vi "WriteReadRegisterLambdaSIM.vi"(4 "period":dbl[](array[numeric]), 5 "VS feedback":dbl[](array[numeric]), 6 "devices 2":refnum<k21>="SLSC-12001-0310EC4F-Mod4", 7 "par 3":T1={"Loop time"={"Loop Rate"=5, "Processor"=-2}, "COM"={"COM IP"="192.168.8.70", "COM port"=30005, "Local port"=5556, "Next_IP 1"=0, "Next_IP 2"=0, "Next_IP 3"=0, "Next_IP 4"=0}, "O2Sensor1"={"Lambda"={"LSU4.2 Lambda"=[], "LSU4.2 Ip"=[], "LSU4.9 Lambda"=[], "LSU4.9 Ip"=[], "LZA03 Lambda"=[], "LZA03 Ip"=[], "LZA08 Lambda"=[], "LZA08 Ip"=[], "Custom Lambda"=[], "Custom Ip"=[]}, "Temp"={"LSU4.2 Temp"=[], "LSU4.2 Ohm"=[], "LSU4.9 Temp"=[], "LSU4.9 Ohm"=[], "LZA03 Temp"=[], "LZA03 Ohm"=[], "LZA08 Temp"=[], "LZA08 Ohm"=[], "Custom Temp"=[], "Custom Ohm"=[]}, "Lambda Type"=0, "PID"={"Ki"=0.0, "Kp"=0.0, "Kd"=0.0, "FeedFW"=0.0}}, "O2Sensor2"={"Lambda"={"LSU4.2 Lambda"=[], "LSU4.2 Ip"=[], "LSU4.9 Lambda"=[], "LSU4.9 Ip"=[], "LZA03 Lambda"=[], "LZA03 Ip"=[], "LZA08 Lambda"=[], "LZA08 Ip"=[], "Custom Lambda"=[], "Custom Ip"=[]}, "Temp"={"LSU4.2 Temp"=[], "LSU4.2 Ohm"=[], "LSU4.9 Temp"=[], "LSU4.9 Ohm"=[], "LZA03 Temp"=[], "LZA03 Ohm"=[], "LZA08 Temp"=[], "LZA08 Ohm"=[], "Custom Temp"=[], "Custom Ohm"=[]}, "Lambda Type"=0, "PID"={"Ki"=0.0, "Kp"=0.0, "Kd"=0.0, "FeedFW"=0.0}}, "O2Sensor3"={"Lambda"={"LSU4.2 Lambda"=[], "LSU4.2 Ip"=[], "LSU4.9 Lambda"=[], "LSU4.9 Ip"=[], "LZA03 Lambda"=[], "LZA03 Ip"=[], "LZA08 Lambda"=[], "LZA08 Ip"=[], "Custom Lambda"=[], "Custom Ip"=[]}, "Temp"={"LSU4.2 Temp"=[], "LSU4.2 Ohm"=[], "LSU4.9 Temp"=[], "LSU4.9 Ohm"=[], "LZA03 Temp"=[], "LZA03 Ohm"=[], "LZA08 Temp"=[], "LZA08 Ohm"=[], "Custom Temp"=[], "Custom Ohm"=[]}, "Lambda Type"=0, "PID"={"Ki"=0.0, "Kp"=0.0, "Kd"=0.0, "FeedFW"=0.0}}, "O2Sensor4"={"Lambda"={"LSU4.2 Lambda"=[], "LSU4.2 Ip"=[], "LSU4.9 Lambda"=[], "LSU4.9 Ip"=[], "LZA03 Lambda"=[], "LZA03 Ip"=[], "LZA08 Lambda"=[], "LZA08 Ip"=[], "Custom Lambda"=[], "Custom Ip"=[]}, "Temp"={"LSU4.2 Temp"=[], "LSU4.2 Ohm"=[], "LSU4.9 Temp"=[], "LSU4.9 Ohm"=[], "LZA03 Temp"=[], "LZA03 Ohm"=[], "LZA08 Temp"=[], "LZA08 Ohm"=[], "Custom Temp"=[], "Custom Ohm"=[]}, "Lambda Type"=0, "PID"={"Ki"=0.0, "Kp"=0.0, "Kd"=0.0, "FeedFW"=0.0}}, "Board"=0, "Mode"=enum."SLSC Mode", "vendor.Num"=4141, "product.Num"=0} {"Board" items=["O2Sim_2ch", "O2Sim_4ch"]; "O2Sensor4"."Lambda Type" items=["LSU4.2", "LSU4.9", "LZA03", "LZA08", "Custom", "[mA]"]; "O2Sensor3"."Lambda Type" items=["LSU4.2", "LSU4.9", "LZA03", "LZA08", "Custom", "[mA]"]; "O2Sensor2"."Lambda Type" items=["LSU4.2", "LSU4.9", "LZA03", "LZA08", "Custom", "[mA]"]; "O2Sensor1"."Lambda Type" items=["LSU4.2", "LSU4.9", "LZA03", "LZA08", "Custom", "[mA]"]}, 8 "error in":errorcluster, 9 "SensorUsed":T3, 10 "VS Control":dbl[](array[numeric]), 11 "session in":refnum<k21>) -> (0 "error out":errorcluster, 2 "VS feedback":dbl[](array[numeric]), 3 "session out":refnum<k21>)   [LabVIEW 2017, in "ALMA_10201-10401_O2SensorSim Engine.lvlib"]
uses:
  ALMA_10201-10401_O2SensorSim Engine.lvlib
  Sensor_used.ctl
  Par.ctl
  LambdaType.ctl
  <vilib>/SLSC/Write Register (U64).vi
  <vilib>/SLSC/Read Register (U64).vi
  <vilib>/SLSC/Set Device Property (I32).vi
  <vilib>/SLSC/SLSC.lvlib
panel:
  out "element":dbl(graph)
  out "#ch_choise":enum16{"O2Sim_2ch", "O2Sim_4ch"}(ring)
  out "com error out":bool
  out "Status":bool[](array[boolean])
  out "Heater DC Indicator":u8[](array[numeric])=[64, 15, 32, 16]
  out "Heater Frequency Indicator2":u8[](array[numeric])=[128, 190, 128, 220]
  out "IP Feedback":dbl[](array[numeric])
  out "Command Cunter Feedback":u8=255
  out "Program Running Cunter":u8=96
  out "IP Feedback 7":dbl[](array[numeric])
  out "Command Cunter Feedback 7":u8=255
  out "Program Running Cunter 7":u8=96
  in  "CommandData 7":u64 format="%048b"
  out "IP Feedback 6":dbl[](array[numeric])
  out "Command Cunter Feedback 6":u8=255
  out "Program Running Cunter 6":u8=96
  in  "CommandData 6":u64 format="%048b"
  out "IP Feedback 5":dbl[](array[numeric])
  out "Command Cunter Feedback 5":u8=255
  out "Program Running Cunter 5":u8=96
  in  "CommandData 5":u64 format="%048b"
  out "IP Feedback 3":dbl[](array[numeric])
  out "Command Cunter Feedback 3":u8=255
  out "Program Running Cunter 3":u8=96
  in  "CommandData 3":u64 format="%048b"
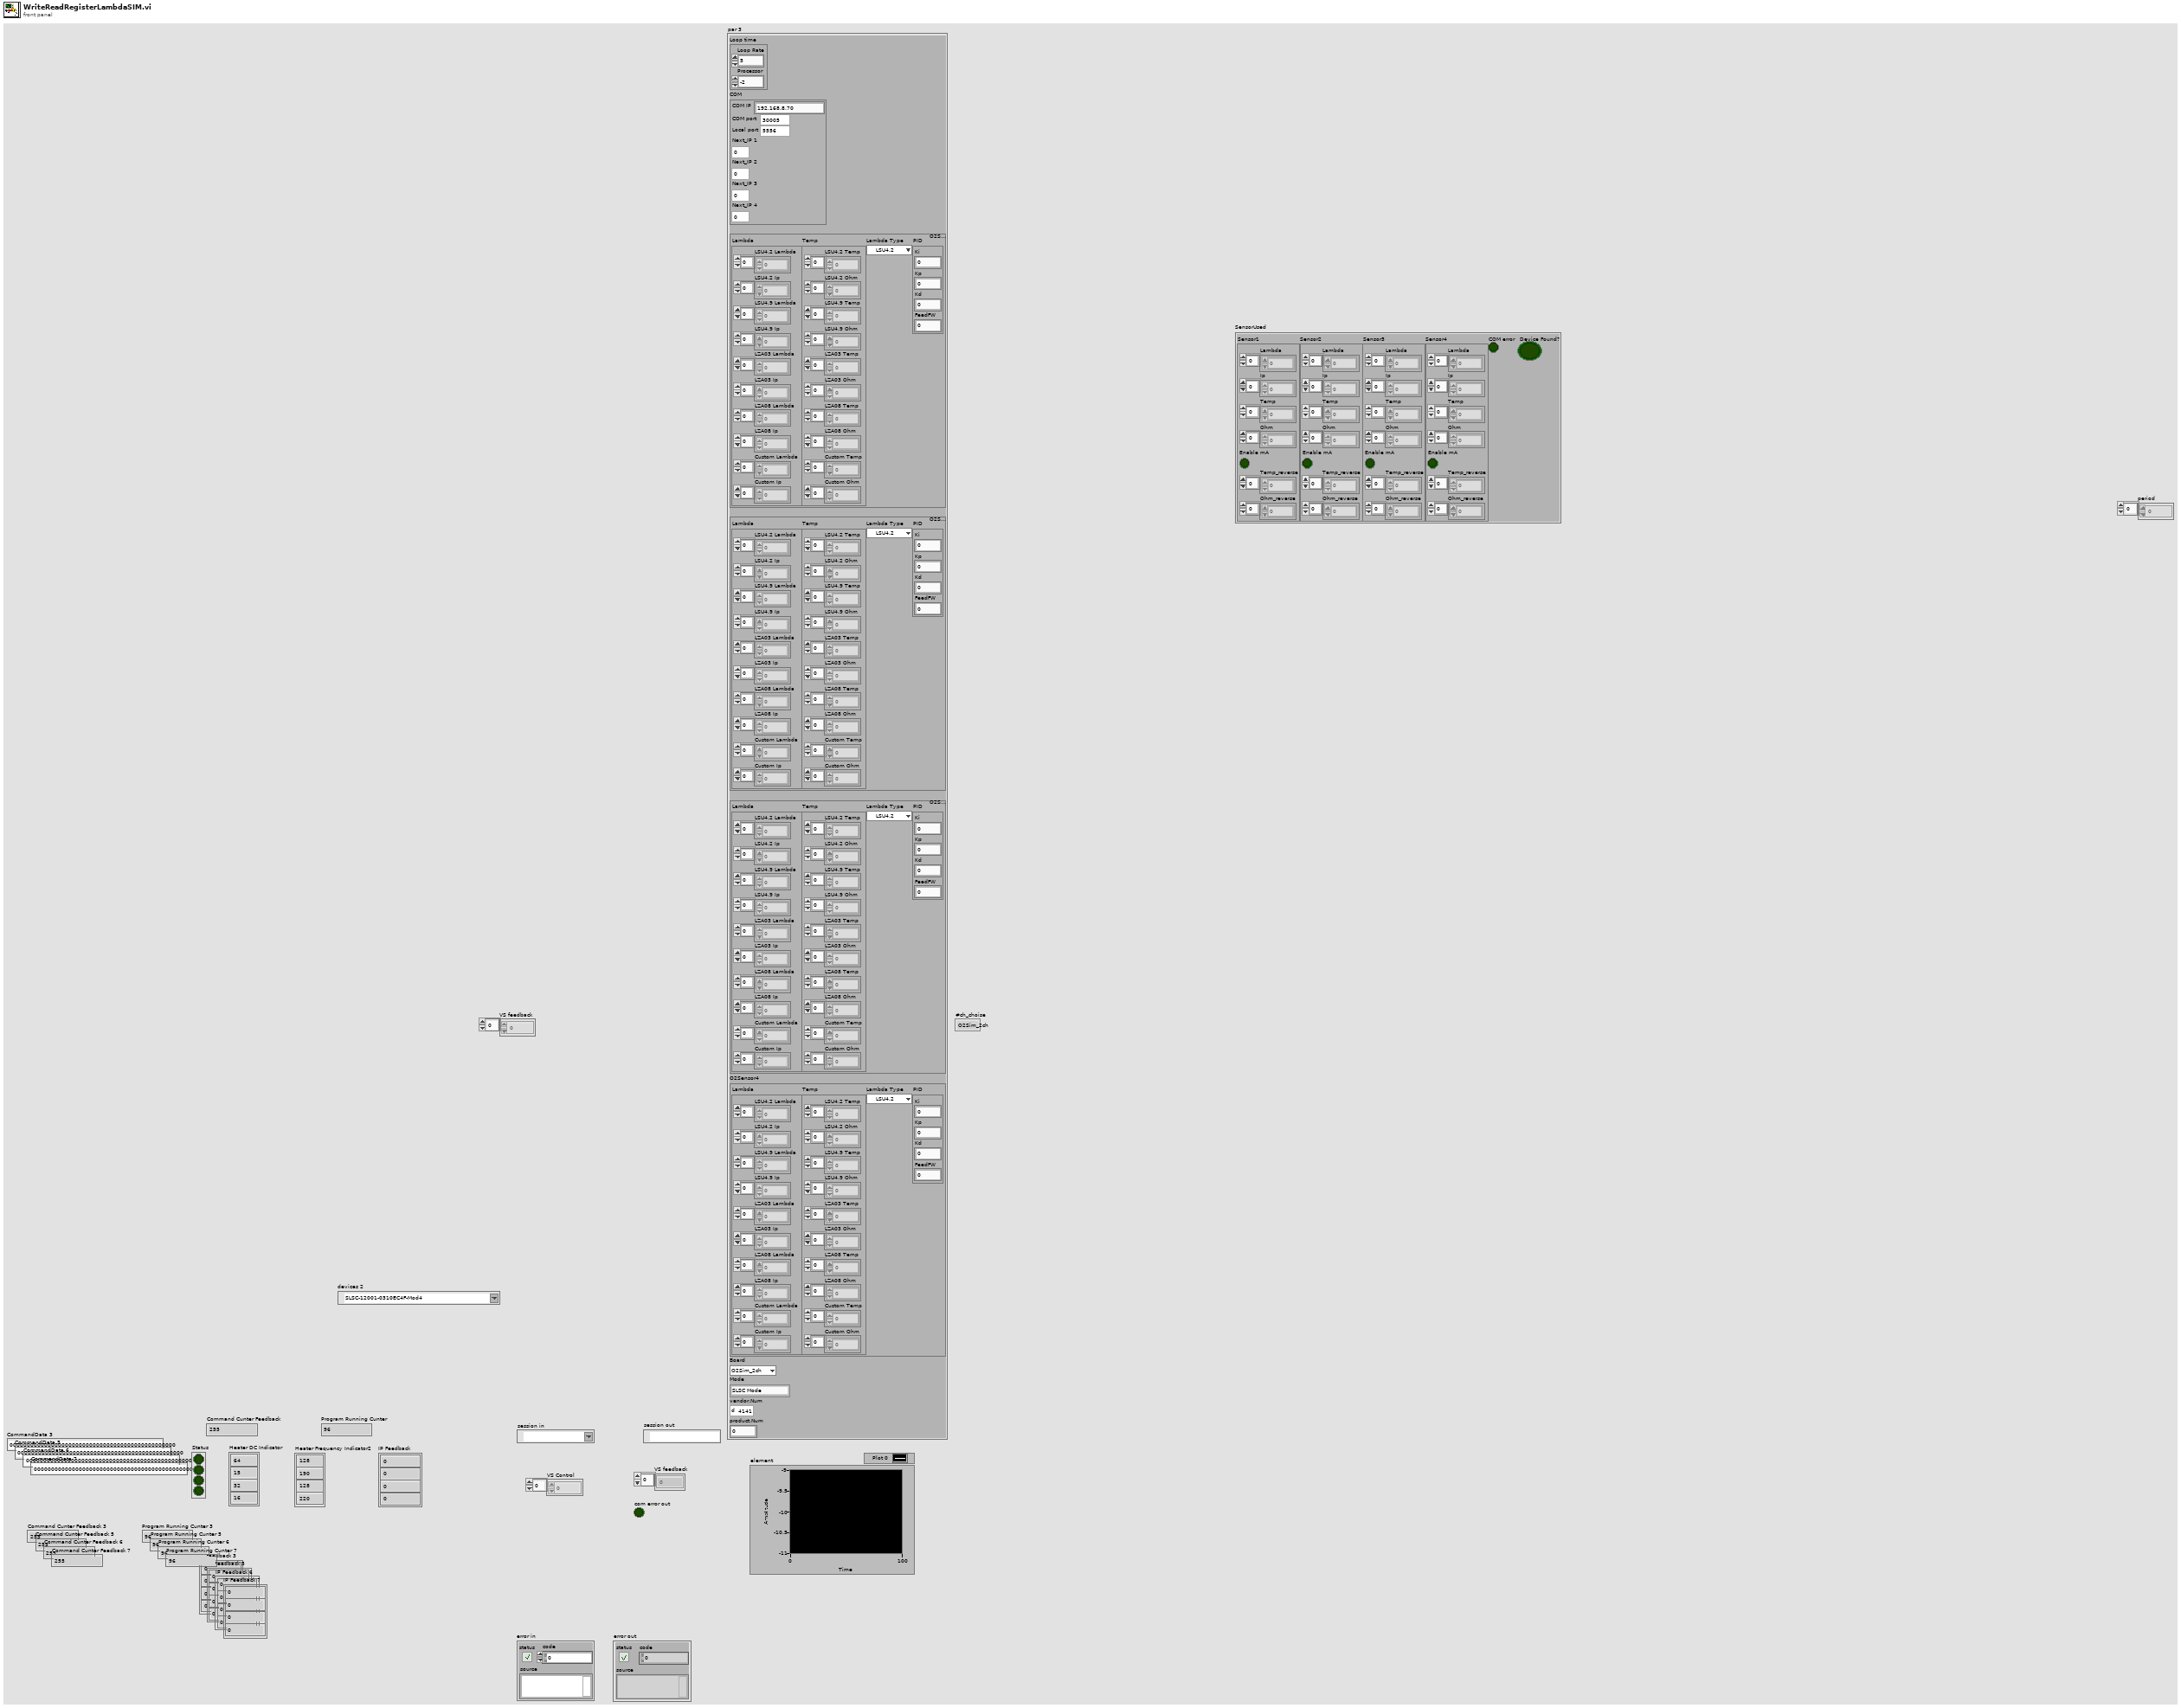
[diagram p1: front panel]
types:
  T1 = typedef "Par.ctl" = cluster{"Loop time":cluster{"Loop Rate":i64, "Processor":i32}, "COM":cluster{"COM IP":string, "COM port":u64, "Local port":u64, "Next_IP 1":u32, "Next_IP 2":u32, "Next_IP 3":u32, "Next_IP 4":u32}, "O2Sensor1":cluster{"Lambda":cluster{"LSU4.2 Lambda":dbl[], "LSU4.2 Ip":dbl[], "LSU4.9 Lambda":dbl[], "LSU4.9 Ip":dbl[], "LZA03 Lambda":dbl[], "LZA03 Ip":dbl[], "LZA08 Lambda":dbl[], "LZA08 Ip":dbl[], "Custom Lambda":dbl[], "Custom Ip":dbl[]}, "Temp":cluster{"LSU4.2 Temp":dbl[], "LSU4.2 Ohm":dbl[], "LSU4.9 Temp":dbl[], "LSU4.9 Ohm":dbl[], "LZA03 Temp":dbl[], "LZA03 Ohm":dbl[], "LZA08 Temp":dbl[], "LZA08 Ohm":dbl[], "Custom Temp":dbl[], "Custom Ohm":dbl[]}, "Lambda Type":T2, "PID":cluster{"Ki":dbl, "Kp":dbl, "Kd":dbl, "FeedFW":dbl}}, "O2Sensor2":cluster{"Lambda":cluster{"LSU4.2 Lambda":dbl[], "LSU4.2 Ip":dbl[], "LSU4.9 Lambda":dbl[], "LSU4.9 Ip":dbl[], "LZA03 Lambda":dbl[], "LZA03 Ip":dbl[], "LZA08 Lambda":dbl[], "LZA08 Ip":dbl[], "Custom Lambda":dbl[], "Custom Ip":dbl[]}, "Temp":cluster{"LSU4.2 Temp":dbl[], "LSU4.2 Ohm":dbl[], "LSU4.9 Temp":dbl[], "LSU4.9 Ohm":dbl[], "LZA03 Temp":dbl[], "LZA03 Ohm":dbl[], "LZA08 Temp":dbl[], "LZA08 Ohm":dbl[], "Custom Temp":dbl[], "Custom Ohm":dbl[]}, "Lambda Type":T2, "PID":cluster{"Ki":dbl, "Kp":dbl, "Kd":dbl, "FeedFW":dbl}}, "O2Sensor3":cluster{"Lambda":cluster{"LSU4.2 Lambda":dbl[], "LSU4.2 Ip":dbl[], "LSU4.9 Lambda":dbl[], "LSU4.9 Ip":dbl[], "LZA03 Lambda":dbl[], "LZA03 Ip":dbl[], "LZA08 Lambda":dbl[], "LZA08 Ip":dbl[], "Custom Lambda":dbl[], "Custom Ip":dbl[]}, "Temp":cluster{"LSU4.2 Temp":dbl[], "LSU4.2 Ohm":dbl[], "LSU4.9 Temp":dbl[], "LSU4.9 Ohm":dbl[], "LZA03 Temp":dbl[], "LZA03 Ohm":dbl[], "LZA08 Temp":dbl[], "LZA08 Ohm":dbl[], "Custom Temp":dbl[], "Custom Ohm":dbl[]}, "Lambda Type":T2, "PID":cluster{"Ki":dbl, "Kp":dbl, "Kd":dbl, "FeedFW":dbl}}, "O2Sensor4":cluster{"Lambda":cluster{"LSU4.2 Lambda":dbl[], "LSU4.2 Ip":dbl[], "LSU4.9 Lambda":dbl[], "LSU4.9 Ip":dbl[], "LZA03 Lambda":dbl[], "LZA03 Ip":dbl[], "LZA08 Lambda":dbl[], "LZA08 Ip":dbl[], "Custom Lambda":dbl[], "Custom Ip":dbl[]}, "Temp":cluster{"LSU4.2 Temp":dbl[], "LSU4.2 Ohm":dbl[], "LSU4.9 Temp":dbl[], "LSU4.9 Ohm":dbl[], "LZA03 Temp":dbl[], "LZA03 Ohm":dbl[], "LZA08 Temp":dbl[], "LZA08 Ohm":dbl[], "Custom Temp":dbl[], "Custom Ohm":dbl[]}, "Lambda Type":T2, "PID":cluster{"Ki":dbl, "Kp":dbl, "Kd":dbl, "FeedFW":dbl}}, "Board":u16, "Mode":enum16{"SLSC Mode", "ANALOG Mode"}, "vendor.Num":u32, "product.Num":u32}
  T2 = typedef "LambdaType.ctl" = u16
  T3 = typedef "ALMA_10201-10401_O2SensorSim Engine.lvlib/Sensor_used.ctl" = cluster{"Sensor1":cluster{"Lambda":dbl[], "Ip":dbl[], "Temp":dbl[], "Ohm":dbl[], "Enable mA":bool, "Temp_reverse":dbl[], "Ohm_reverse":dbl[]}, "Sensor2":cluster{"Lambda":dbl[], "Ip":dbl[], "Temp":dbl[], "Ohm":dbl[], "Enable mA":bool, "Temp_reverse":dbl[], "Ohm_reverse":dbl[]}, "Sensor3":cluster{"Lambda":dbl[], "Ip":dbl[], "Temp":dbl[], "Ohm":dbl[], "Enable mA":bool, "Temp_reverse":dbl[], "Ohm_reverse":dbl[]}, "Sensor4":cluster{"Lambda":dbl[], "Ip":dbl[], "Temp":dbl[], "Ohm":dbl[], "Enable mA":bool, "Temp_reverse":dbl[], "Ohm_reverse":dbl[]}, "COM error":bool, "Device Found?":bool}
  T4 = cluster{"Lambda":dbl[], "Ip":dbl[], "Temp":dbl[], "Ohm":dbl[], "Enable mA":bool, "Temp_reverse":dbl[], "Ohm_reverse":dbl[]}
  T5 = cluster{"Lambda":dbl[], "Ip":dbl[], "Temp":dbl[], "Ohm":dbl[], "Enable mA":bool, "Temp_reverse":dbl[], "Ohm_reverse":dbl[]}[]
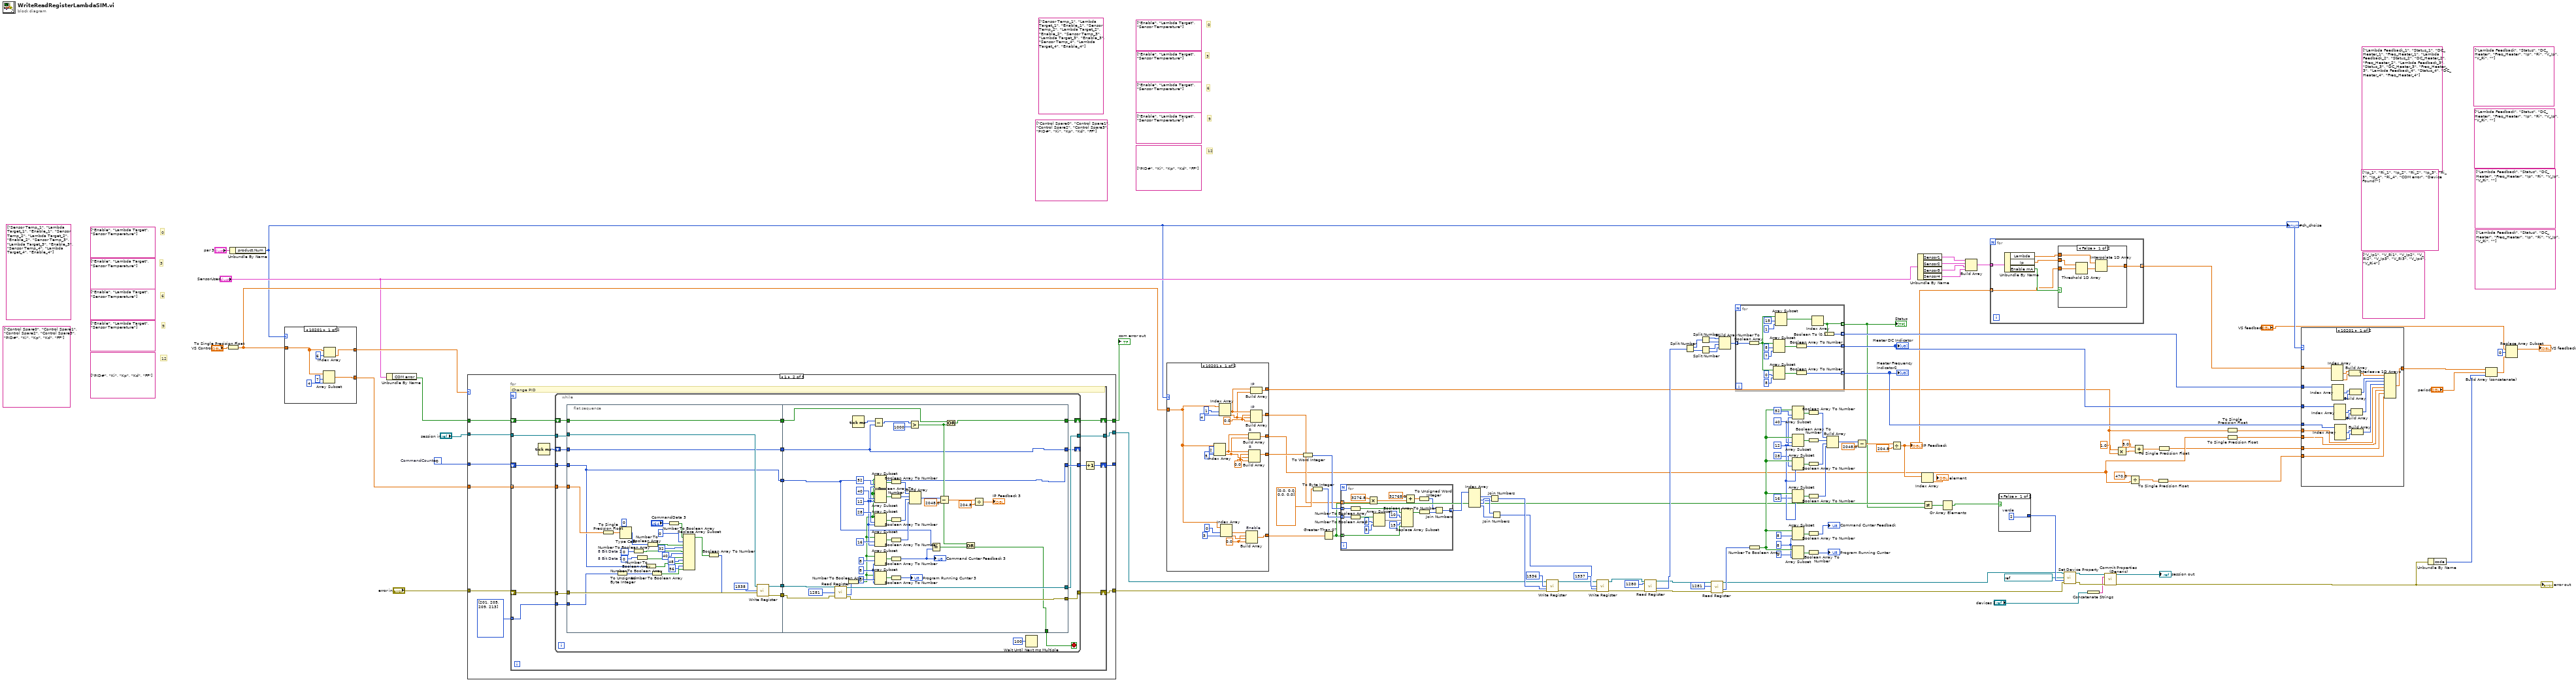
[diagram p0: block diagram]
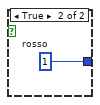
[diagram p2: hidden frame]
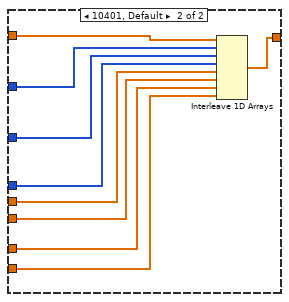
[diagram p3: hidden frame]
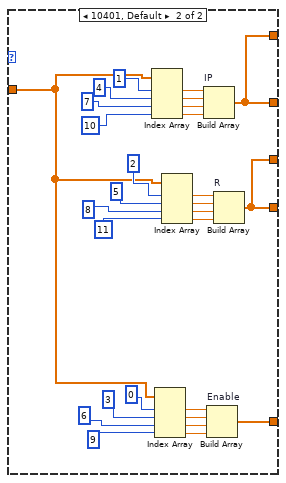
[diagram p4: hidden frame]
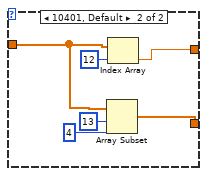
[diagram p5: hidden frame]
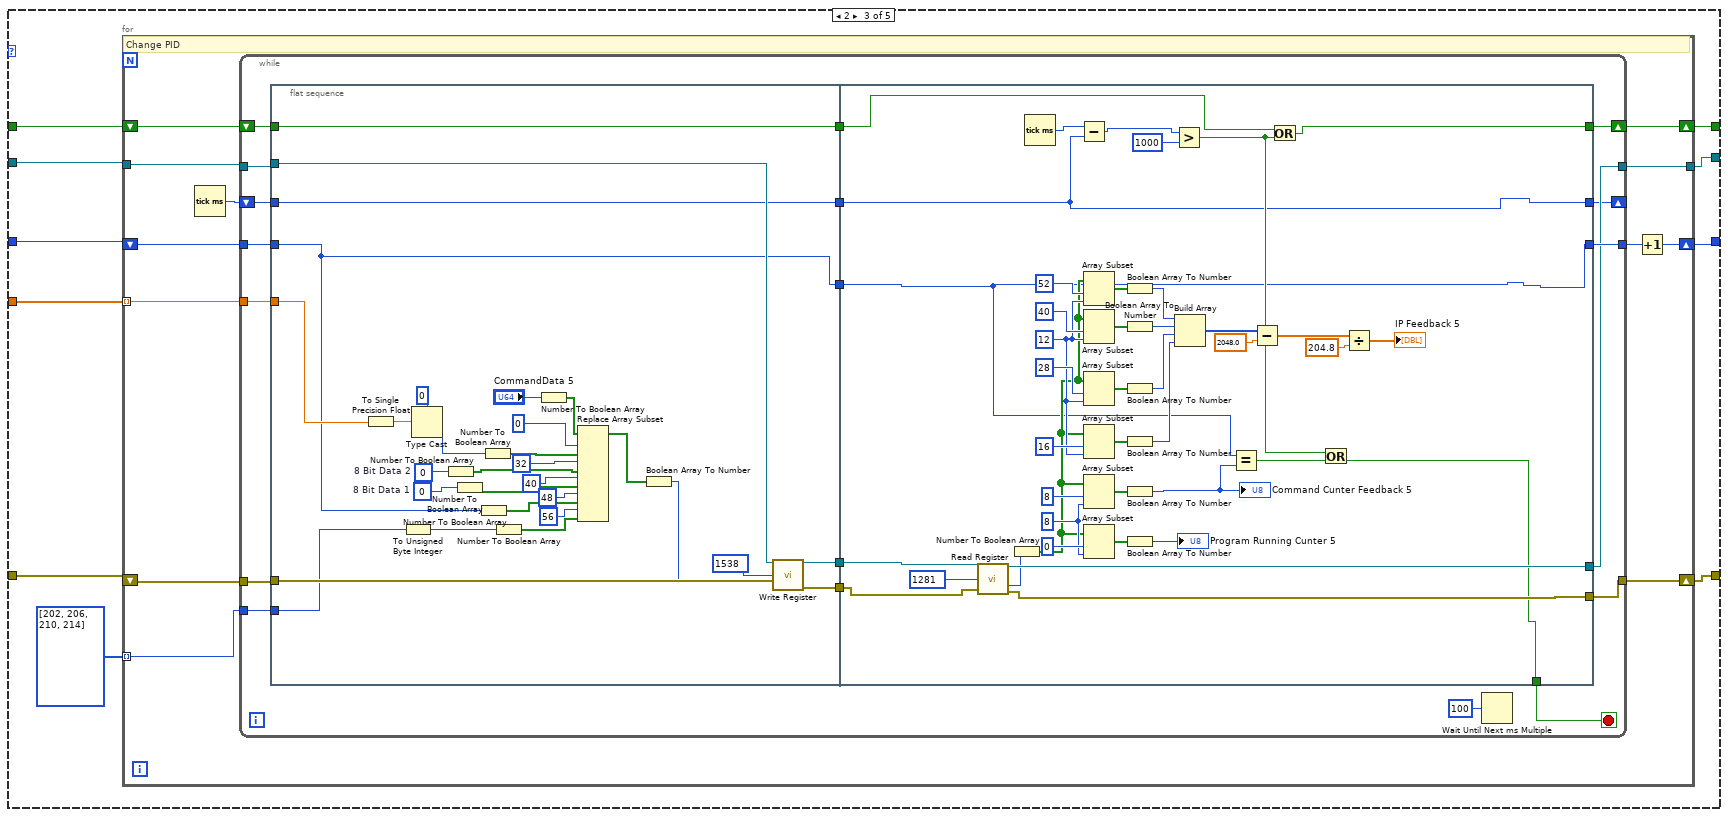
[diagram p8: hidden frame]
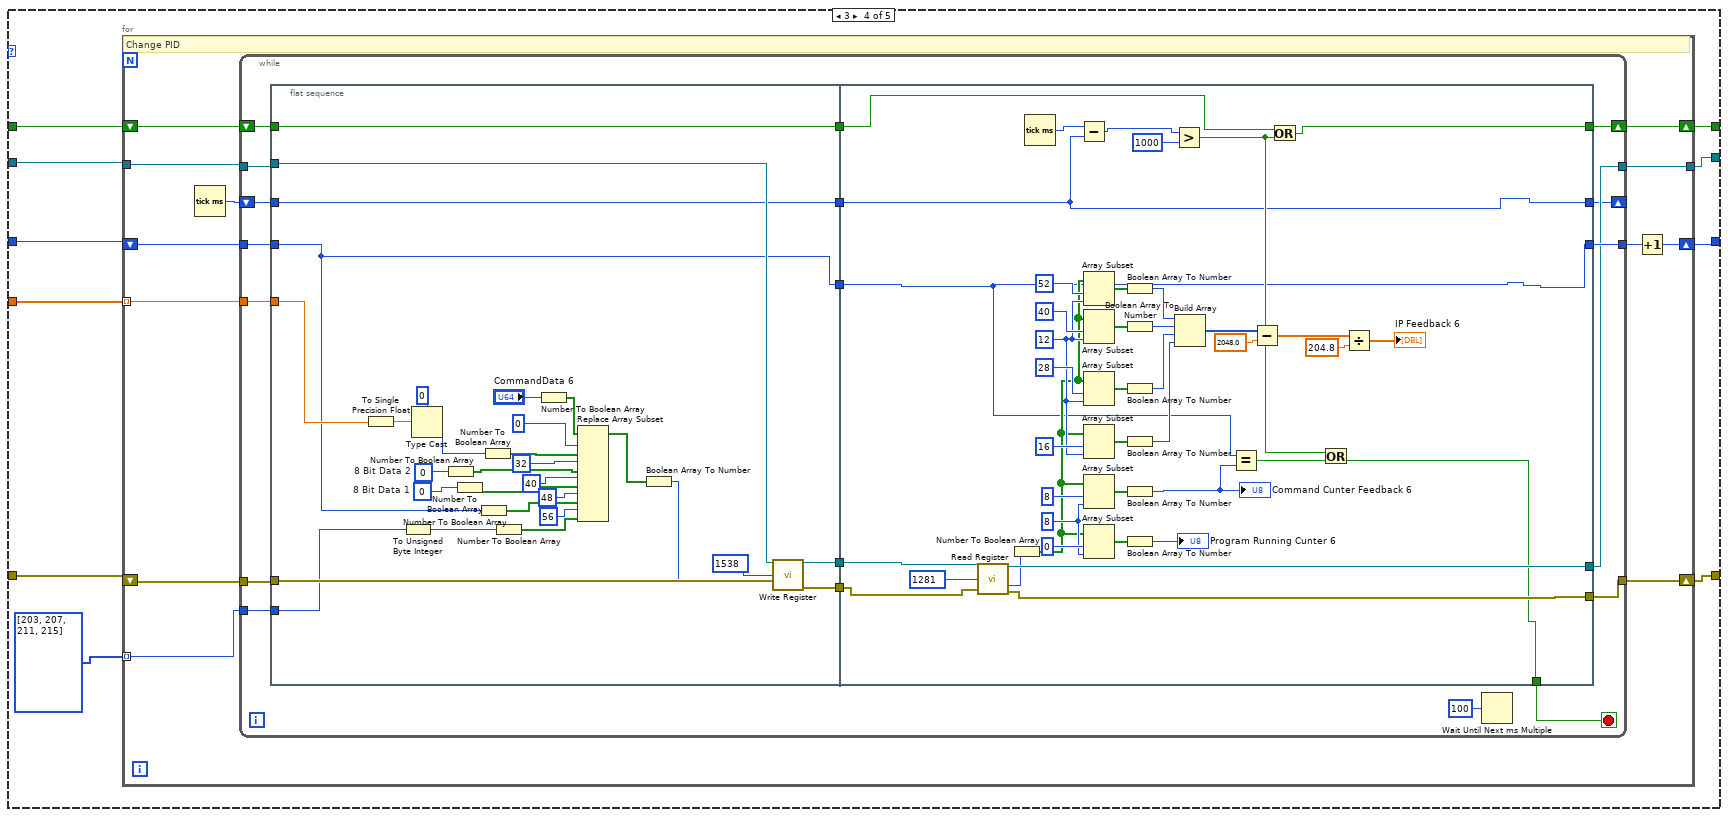
[diagram p9: hidden frame]
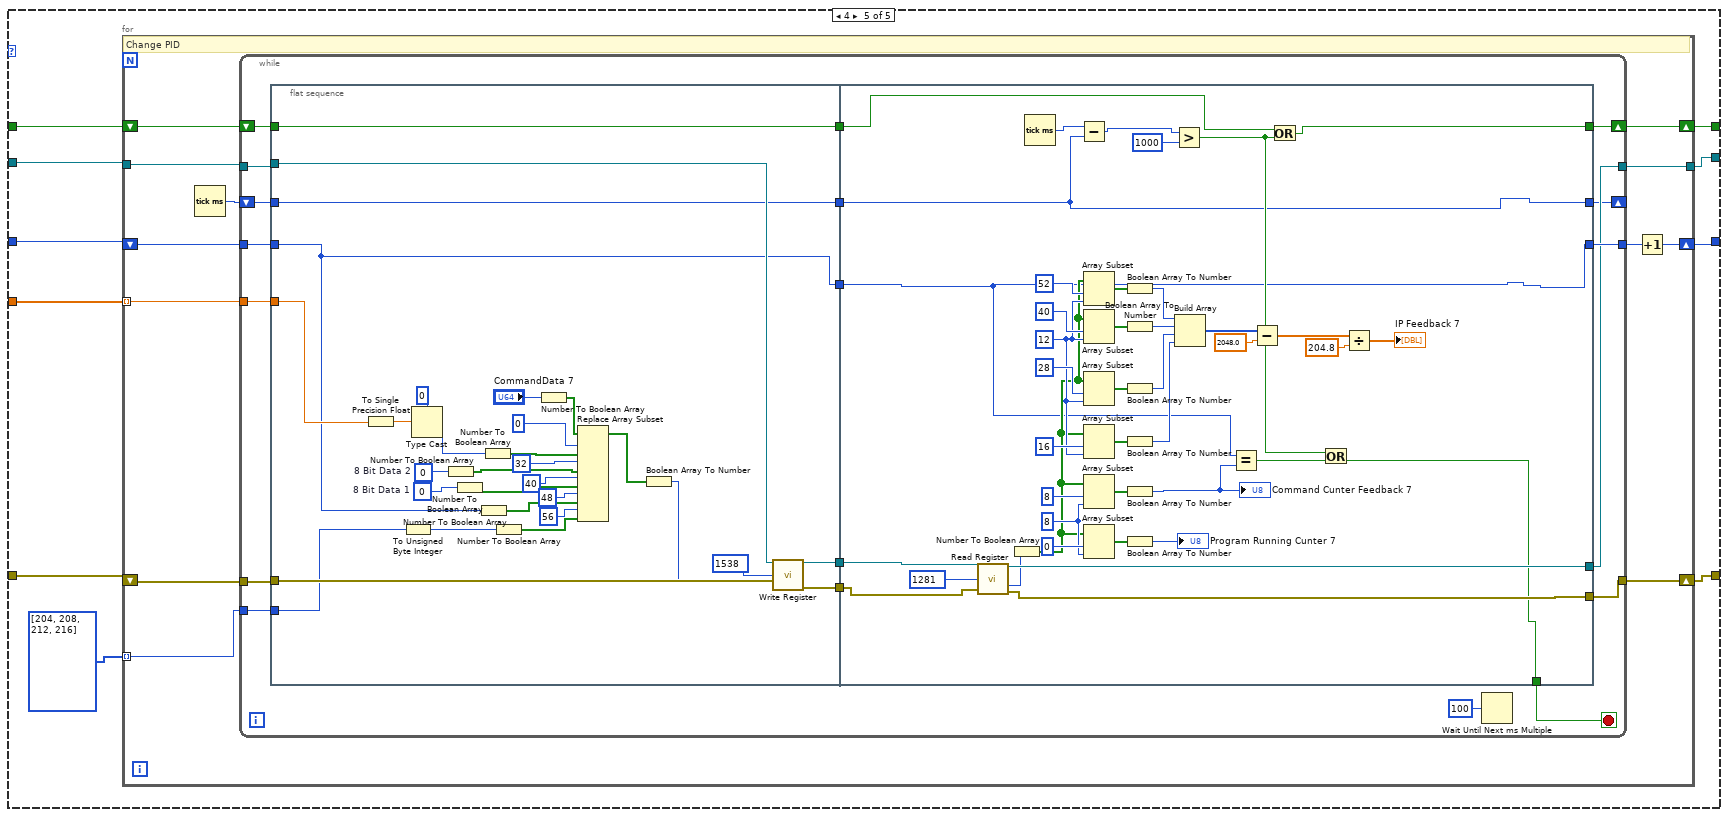
[diagram p10: hidden frame]
diagram:
  (unwired) string[] ["PID#", "Ki", "Kp", "Kd", "FF"] ("O2SensoSim Setpoint 2")
  (unwired) string[] ["Enable", "Lambda Target", "Sensor Temperature"] ("O2SensoSim Setpoint 2")
  (unwired) string[] ["Enable", "Lambda Target", "Sensor Temperature"] ("O2SensoSim Setpoint 2")
  (unwired) string[] ["Enable", "Lambda Target", "Sensor Temperature"] ("O2SensoSim Setpoint 2")
  (unwired) string[] ["Enable", "Lambda Target", "Sensor Temperature"] ("O2SensoSim Setpoint 2")
  (unwired) string[] ["Lambda Feedback", "Status", "DC_Heater", "Freq_Heater", "Ip", "Ri", "V_Ip", "V_Ri", ""] ("O2SensoSim Feedback 4")
  (unwired) string[] ["Lambda Feedback", "Status", "DC_Heater", "Freq_Heater", "Ip", "Ri", "V_Ip", "V_Ri", ""] ("O2SensoSim Feedback 4")
  (unwired) string[] ["Lambda Feedback", "Status", "DC_Heater", "Freq_Heater", "Ip", "Ri", "V_Ip", "V_Ri", ""] ("O2SensoSim Feedback 4")
  (unwired) string[] ["Lambda Feedback", "Status", "DC_Heater", "Freq_Heater", "Ip", "Ri", "V_Ip", "V_Ri", ""] ("O2SensoSim Feedback 4")
  (unwired) string[] ["PID#", "Ki", "Kp", "Kd", "FF"] ("O2SensoSim Setpoint 2")
  (unwired) string[] ["Enable", "Lambda Target", "Sensor Temperature"] ("O2SensoSim Setpoint 2")
  (unwired) string[] ["Enable", "Lambda Target", "Sensor Temperature"] ("O2SensoSim Setpoint 2")
  (unwired) string[] ["Enable", "Lambda Target", "Sensor Temperature"] ("O2SensoSim Setpoint 2")
  (unwired) string[] ["Enable", "Lambda Target", "Sensor Temperature"] ("O2SensoSim Setpoint 2")
  (unwired) string[] ["V_Ip1", "V_Ri1", "V_Ip2", "V_Ri2", "V_Ip3", "V_Ri3", "V_Ip4", "V_Ri4"] ("O2SensoSim Feedback 3")
  (unwired) string[] ["Control Spare0", "Control Spare1", "Control Spare2", "Control Spare3", "PID#", "Ki", "Kp", "Kd", "FF"] ("Additional Control")
  (unwired) string[] ["Sensor Temp_1", "Lambda Target_1", "Enable_1", "Sensor Temp_2", "Lambda Target_2", "Enable_2", "Sensor Temp_3", "Lambda Target_3", "Enable_3", "Sensor Temp_4", "Lambda Target_4", "Enable_4"] ("O2SensoSim Setpoint 2")
  w78 = 8 ("length")
  w77 = 12 ("length")
  (unwired) string[] ["Control Spare0", "Control Spare1", "Control Spare2", "Control Spare3", "PID#", "Ki", "Kp", "Kd", "FF"] ("Additional Control")
  (unwired) string[] ["Ip_1", "Ri_1", "Ip_2", "Ri_2", "Ip_3", "Ri_3", "Ip_4", "Ri_4", "COM error", "Device Found?"] ("O2SensoSim Feedback 3")
  (unwired) string[] ["Lambda Feedback_1", "Status_1", "DC_Heater_1", "Freq_Heater_1", "Lambda Feedback_2", "Status_2", "DC_Heater_2", "Freq_Heater_2", "Lambda Feedback_3", "Status_3", "DC_Heater_3", "Freq_Heater_3", "Lambda Feedback_4", "Status_4", "DC_Heater_4", "Freq_Heater_4"] ("O2SensoSim Feedback 4")
  (unwired) string[] ["Sensor Temp_1", "Lambda Target_1", "Enable_1", "Sensor Temp_2", "Lambda Target_2", "Enable_2", "Sensor Temp_3", "Lambda Target_3", "Enable_3", "Sensor Temp_4", "Lambda Target_4", "Enable_4"] ("O2SensoSim Setpoint 2")
  w112 = u8 0  # CommandCounter
  # "12"
  # "9"
  # "6"
  # "3"
  # "0"
  # "12"
  # "9"
  # "6"
  # "3"
  # "0"
  n1 = To Single Precision Float(number="VS Control") -> (single precision float=w56:sgl[])
  n2 = Unbundle By Name("par 3") -> ("product.Num"=w42:u32)
  "#ch_choise" <- w42
  n3 = case shown="10201" w42 {
    tunnel: [w117 w126] -> w111
    tunnel: [w116 w123] -> w110
    tunnel: w56 -> [w118 w122]
    frame 10201 {
      n4 = Array Subset(array=w118, index=7, length=4) -> (w116:sgl[])
      n5 = Index Array(array=w118, index=6) -> (element=w117:sgl)
    }
    frame 10401, Default {
      n6 = Array Subset(array=w122, index=13, length=4) -> (w123:sgl[])
      n7 = Index Array(array=w122, index=12) -> (element=w126:sgl)
    }
  }
  n8 = Unbundle By Name("SensorUsed") -> ("COM error"=w45:bool)
  n9 = case shown="1" w111 {
    tunnel: "error in" -> [w128 w141 w254 w367 w480]
    tunnel: w45 -> [w131 w140 w253 w366 w479]
    tunnel: "session in" -> [w130 w139 w252 w365 w478]
    tunnel: w112 -> [w129 w138 w251 w364 w477]
    tunnel: [w131 w136 w248 w362 w475] -> w51
    tunnel: [w130 w135 w247 w361 w474] -> w58
    tunnel: [w129 w134 w246 w360 w473] -> _
    tunnel: [w128 w133 w245 w358 w471] -> w59
    tunnel: w110 -> [_ w137 w250 w363 w476]
    frame 0, Default {
    }
    frame 1 {
      n10 = for {
        tunnel: w139 -> [w153]
        tunnel: w137 -> [w152] mode=indexing
        shift-right: [w144] -> w134
        shift-left: w138 -> [w151]
        shift-right: [w149] -> w133
        shift-left: w141 -> [w143]
        tunnel: [w148] -> w135
        shift-right: [w145] -> w136
        shift-left: w140 -> [w147]
        tunnel: u8[] [201, 205, 209, 213] -> [w142] mode=indexing
        # "Change PID"
        n11 = Tick Count (ms)() -> (millisecond timer value=w146:u32)
        n12 = while {
          tunnel: w152 -> [w168]
          tunnel: w151 -> [w167]
          tunnel: [w166] -> w150
          tunnel: [w165] -> w149
          tunnel: w143 -> [w164]
          shift-right: [w158] -> _
          shift-left: w146 -> [w161]
          shift-right: [w156] -> w145
          shift-left: w147 -> [w162]
          tunnel: w142 -> [w155]
          tunnel: w153 -> [w169]
          tunnel: [w163] -> w148
          stop <- w159 stop-if-true
          n13 = flat-sequence {
            tunnel: w164 -> [w201]
            tunnel: w169 -> [w200]
            tunnel: [w180] -> w172
            tunnel: [w179] -> w171
            tunnel: [w177] -> w170
            tunnel: w168 -> [w178]
            tunnel: w167 -> [w177]
            tunnel: w162 -> [w175]
            tunnel: w161 -> [w176]
            tunnel: [w176] -> w160
            tunnel: [w175] -> w157
            tunnel: w155 -> [w174]
            tunnel: w172 -> [w244]
            tunnel: w171 -> [w243]
            tunnel: w170 -> [w204]
            tunnel: [w204] -> w166
            tunnel: [w242] -> w165
            tunnel: [w241] -> w163
            tunnel: w160 -> [w203]
            tunnel: [w209] -> w159
            tunnel: [w203] -> w158
            tunnel: w157 -> [w207]
            tunnel: [w205] -> w156
            frame #0 {
              w183 = u8 0  # 8 Bit Data 2
              w184 = u8 0  # 8 Bit Data 1
              n14 = To Single Precision Float(number=w178) -> (single precision float=w192:sgl)
              n15 = To Unsigned Byte Integer(number=w174) -> (unsigned 8bit integer=w173:u8)
              n16 = Type Cast(type=u32 0 ("index"), x=w192) -> (*(type *) &x=w185:u32)
              n17 = Number To Boolean Array(number=w183) -> (Boolean array=w181:bool[])
              n18 = Number To Boolean Array(number=w184) -> (Boolean array=w182:bool[])
              n19 = Number To Boolean Array(number=w177) -> (Boolean array=w187:bool[])
              n20 = Number To Boolean Array(number=w185) -> (Boolean array=w186:bool[])
              n21 = Number To Boolean Array(number=w173) -> (Boolean array=w196:bool[])
              n22 = Number To Boolean Array(number="CommandData 3") -> (Boolean array=w198:bool[])
              n23 = Replace Array Subset(array=w198, new element #1=w186, index #1=0 ("index"), new element #2=w181, index #2=32 ("index"), new element #3=w182, index #3=40 ("index"), new element #4=w187, index #4=48 ("index"), new element #5=w196, index #5=56 ("index")) -> (w197:bool[])
              n24 = Boolean Array To Number(Boolean array=w197) -> (number=w193:u64)
              n25 = call-poly <vilib>:"Write Register.vi"("session in"=w200, "register address"=u32 1538, "data"=w193, "error in (no error)"=w201) -> ("session out"=w179:refnum<k21>, "error out"=w180:errorcluster)  [unwired: 8 in, 2 out]
            }
            frame #1 {
              w232 = 8 ("length")
              w233 = 12 ("length")
              n26 = call-poly <vilib>:"Read Register.vi"("session in"=w243, "register address"=u32 1281 ("y"), "error in (no error)"=w244) -> ("session out"=w241:refnum<k21>, "data out"=w214:u64, "error out"=w242:errorcluster)  [unwired: 8 in, 2 out]
              n27 = Number To Boolean Array(number=w214) -> (Boolean array=w227:bool[])
              n28 = Tick Count (ms)() -> (millisecond timer value=w208:u32)
              n29 = Subtract(x=w208, y=w203) -> (x-y=w211:u32)
              n30 = Array Subset(array=w227, index=52, length=w233) -> (w228:bool[])
              n31 = Array Subset(array=w227, index=40, length=w233) -> (w226:bool[])
              n32 = Array Subset(array=w227, index=28, length=w233) -> (w225:bool[])
              n33 = Array Subset(array=w227, index=16, length=w233) -> (w224:bool[])
              n34 = Array Subset(array=w227, index=8, length=w232) -> (w223:bool[])
              n35 = Array Subset(array=w227, index=0, length=w232) -> (w222:bool[])
              n36 = Boolean Array To Number(Boolean array=w228) -> (number=w216:u16)
              n37 = Boolean Array To Number(Boolean array=w226) -> (number=w231:u16)
              n38 = Boolean Array To Number(Boolean array=w225) -> (number=w230:u16)
              n39 = Boolean Array To Number(Boolean array=w224) -> (number=w229:u16)
              n40 = Boolean Array To Number(Boolean array=w223) -> (number=w213:u8)
              "Command Cunter Feedback 3" <- w213
              n41 = Boolean Array To Number(Boolean array=w222) -> (number=→"Program Running Cunter 3":u8)
              n42 = Greater?(x=w211, y=u32 1000) -> (0:w206:bool)
              n43 = Build Array(w216, w231, w230, w229) -> (w217:u16[])
              n44 = Equal?(x=w204, y=w213) -> (x = y?=w212:bool)
              n45 = Subtract(x=w217, y=2048.0) -> (x-y=w220:dbl[])
              n46 = Or(x=w207, y=w206) -> (x .or. y?=w205:bool)
              n47 = Or(x=w206, y=w212) -> (x .or. y?=w209:bool)
              n48 = Divide(x=w220, y=204.8) -> (x/y=→"IP Feedback 3":dbl[])
            }
          }
          n49 = Wait Until Next ms Multiple(millisecond multiple=u32 100) -> ()  [unwired: 1 out]
        }
        n50 = Increment(x=w150) -> (x+1=w144:u8)
      }
    }
    frame 2 {
      n51 = for {
        tunnel: w252 -> [w266]
        tunnel: w250 -> [w265] mode=indexing
        shift-right: [w256] -> w246
        shift-left: w251 -> [w264]
        shift-right: [w262] -> w245
        shift-left: w254 -> [w261]
        tunnel: [w260] -> w247
        shift-right: [w257] -> w248
        shift-left: w253 -> [w259]
        tunnel: u8[] [202, 206, 210, 214] -> [w255] mode=indexing
        # "Change PID"
        n52 = Tick Count (ms)() -> (millisecond timer value=w258:u32)
        n53 = while {
          tunnel: w265 -> [w281]
          tunnel: w264 -> [w280]
          tunnel: [w279] -> w263
          tunnel: [w278] -> w262
          tunnel: w261 -> [w277]
          shift-right: [w271] -> _
          shift-left: w258 -> [w274]
          shift-right: [w269] -> w257
          shift-left: w259 -> [w275]
          tunnel: w255 -> [w268]
          tunnel: w266 -> [w282]
          tunnel: [w276] -> w260
          stop <- w272 stop-if-true
          n54 = flat-sequence {
            tunnel: w277 -> [w314]
            tunnel: w282 -> [w313]
            tunnel: [w293] -> w285
            tunnel: [w292] -> w284
            tunnel: [w290] -> w283
            tunnel: w281 -> [w291]
            tunnel: w280 -> [w290]
            tunnel: w275 -> [w288]
            tunnel: w274 -> [w289]
            tunnel: [w289] -> w273
            tunnel: [w288] -> w270
            tunnel: w268 -> [w287]
            tunnel: w285 -> [w357]
            tunnel: w284 -> [w356]
            tunnel: w283 -> [w317]
            tunnel: [w317] -> w279
            tunnel: [w355] -> w278
            tunnel: [w354] -> w276
            tunnel: w273 -> [w316]
            tunnel: [w322] -> w272
            tunnel: [w316] -> w271
            tunnel: w270 -> [w320]
            tunnel: [w318] -> w269
            frame #0 {
              w296 = u8 0  # 8 Bit Data 2
              w297 = u8 0  # 8 Bit Data 1
              n55 = To Single Precision Float(number=w291) -> (single precision float=w305:sgl)
              n56 = To Unsigned Byte Integer(number=w287) -> (unsigned 8bit integer=w286:u8)
              n57 = Type Cast(type=u32 0 ("index"), x=w305) -> (*(type *) &x=w298:u32)
              n58 = Number To Boolean Array(number=w296) -> (Boolean array=w294:bool[])
              n59 = Number To Boolean Array(number=w297) -> (Boolean array=w295:bool[])
              n60 = Number To Boolean Array(number=w290) -> (Boolean array=w300:bool[])
              n61 = Number To Boolean Array(number=w298) -> (Boolean array=w299:bool[])
              n62 = Number To Boolean Array(number=w286) -> (Boolean array=w309:bool[])
              n63 = Number To Boolean Array(number="CommandData 5") -> (Boolean array=w311:bool[])
              n64 = Replace Array Subset(array=w311, new element #1=w299, index #1=0 ("index"), new element #2=w294, index #2=32 ("index"), new element #3=w295, index #3=40 ("index"), new element #4=w300, index #4=48 ("index"), new element #5=w309, index #5=56 ("index")) -> (w310:bool[])
              n65 = Boolean Array To Number(Boolean array=w310) -> (number=w306:u64)
              n66 = call-poly <vilib>:"Write Register.vi"("session in"=w313, "register address"=u32 1538, "data"=w306, "error in (no error)"=w314) -> ("session out"=w292:refnum<k21>, "error out"=w293:errorcluster)  [unwired: 8 in, 2 out]
            }
            frame #1 {
              w345 = 8 ("length")
              w346 = 12 ("length")
              n67 = call-poly <vilib>:"Read Register.vi"("session in"=w356, "register address"=u32 1281 ("y"), "error in (no error)"=w357) -> ("session out"=w354:refnum<k21>, "data out"=w327:u64, "error out"=w355:errorcluster)  [unwired: 8 in, 2 out]
              n68 = Number To Boolean Array(number=w327) -> (Boolean array=w340:bool[])
              n69 = Tick Count (ms)() -> (millisecond timer value=w321:u32)
              n70 = Subtract(x=w321, y=w316) -> (x-y=w324:u32)
              n71 = Array Subset(array=w340, index=52, length=w346) -> (w341:bool[])
              n72 = Array Subset(array=w340, index=40, length=w346) -> (w339:bool[])
              n73 = Array Subset(array=w340, index=28, length=w346) -> (w338:bool[])
              n74 = Array Subset(array=w340, index=16, length=w346) -> (w337:bool[])
              n75 = Array Subset(array=w340, index=8, length=w345) -> (w336:bool[])
              n76 = Array Subset(array=w340, index=0, length=w345) -> (w335:bool[])
              n77 = Boolean Array To Number(Boolean array=w341) -> (number=w329:u16)
              n78 = Boolean Array To Number(Boolean array=w339) -> (number=w344:u16)
              n79 = Boolean Array To Number(Boolean array=w338) -> (number=w343:u16)
              n80 = Boolean Array To Number(Boolean array=w337) -> (number=w342:u16)
              n81 = Boolean Array To Number(Boolean array=w336) -> (number=w326:u8)
              "Command Cunter Feedback 5" <- w326
              n82 = Boolean Array To Number(Boolean array=w335) -> (number=→"Program Running Cunter 5":u8)
              n83 = Greater?(x=w324, y=u32 1000) -> (0:w319:bool)
              n84 = Build Array(w329, w344, w343, w342) -> (w330:u16[])
              n85 = Equal?(x=w317, y=w326) -> (x = y?=w325:bool)
              n86 = Subtract(x=w330, y=2048.0) -> (x-y=w333:dbl[])
              n87 = Or(x=w320, y=w319) -> (x .or. y?=w318:bool)
              n88 = Or(x=w319, y=w325) -> (x .or. y?=w322:bool)
              n89 = Divide(x=w333, y=204.8) -> (x/y=→"IP Feedback 5":dbl[])
            }
          }
          n90 = Wait Until Next ms Multiple(millisecond multiple=u32 100) -> ()  [unwired: 1 out]
        }
        n91 = Increment(x=w263) -> (x+1=w256:u8)
      }
    }
    frame 3 {
      n92 = for {
        tunnel: w365 -> [w379]
        tunnel: w363 -> [w378] mode=indexing
        shift-right: [w369] -> w360
        shift-left: w364 -> [w377]
        shift-right: [w375] -> w358
        shift-left: w367 -> [w374]
        tunnel: [w373] -> w361
        shift-right: [w370] -> w362
        shift-left: w366 -> [w372]
        tunnel: u8[] [203, 207, 211, 215] -> [w368] mode=indexing
        # "Change PID"
        n93 = Tick Count (ms)() -> (millisecond timer value=w371:u32)
        n94 = while {
          tunnel: w378 -> [w394]
          tunnel: w377 -> [w393]
          tunnel: [w392] -> w376
          tunnel: [w391] -> w375
          tunnel: w374 -> [w390]
          shift-right: [w384] -> _
          shift-left: w371 -> [w387]
          shift-right: [w382] -> w370
          shift-left: w372 -> [w388]
          tunnel: w368 -> [w381]
          tunnel: w379 -> [w395]
          tunnel: [w389] -> w373
          stop <- w385 stop-if-true
          n95 = flat-sequence {
            tunnel: w390 -> [w427]
            tunnel: w395 -> [w426]
            tunnel: [w406] -> w398
            tunnel: [w405] -> w397
            tunnel: [w403] -> w396
            tunnel: w394 -> [w404]
            tunnel: w393 -> [w403]
            tunnel: w388 -> [w401]
            tunnel: w387 -> [w402]
            tunnel: [w402] -> w386
            tunnel: [w401] -> w383
            tunnel: w381 -> [w400]
            tunnel: w398 -> [w470]
            tunnel: w397 -> [w469]
            tunnel: w396 -> [w430]
            tunnel: [w430] -> w392
            tunnel: [w468] -> w391
            tunnel: [w467] -> w389
            tunnel: w386 -> [w429]
            tunnel: [w435] -> w385
            tunnel: [w429] -> w384
            tunnel: w383 -> [w433]
            tunnel: [w431] -> w382
            frame #0 {
              w409 = u8 0  # 8 Bit Data 2
              w410 = u8 0  # 8 Bit Data 1
              n96 = To Single Precision Float(number=w404) -> (single precision float=w418:sgl)
              n97 = To Unsigned Byte Integer(number=w400) -> (unsigned 8bit integer=w399:u8)
              n98 = Type Cast(type=u32 0 ("index"), x=w418) -> (*(type *) &x=w411:u32)
              n99 = Number To Boolean Array(number=w409) -> (Boolean array=w407:bool[])
              n100 = Number To Boolean Array(number=w410) -> (Boolean array=w408:bool[])
              n101 = Number To Boolean Array(number=w403) -> (Boolean array=w413:bool[])
              n102 = Number To Boolean Array(number=w411) -> (Boolean array=w412:bool[])
              n103 = Number To Boolean Array(number=w399) -> (Boolean array=w422:bool[])
              n104 = Number To Boolean Array(number="CommandData 6") -> (Boolean array=w424:bool[])
              n105 = Replace Array Subset(array=w424, new element #1=w412, index #1=0 ("index"), new element #2=w407, index #2=32 ("index"), new element #3=w408, index #3=40 ("index"), new element #4=w413, index #4=48 ("index"), new element #5=w422, index #5=56 ("index")) -> (w423:bool[])
              n106 = Boolean Array To Number(Boolean array=w423) -> (number=w419:u64)
              n107 = call-poly <vilib>:"Write Register.vi"("session in"=w426, "register address"=u32 1538, "data"=w419, "error in (no error)"=w427) -> ("session out"=w405:refnum<k21>, "error out"=w406:errorcluster)  [unwired: 8 in, 2 out]
            }
            frame #1 {
              w458 = 8 ("length")
              w459 = 12 ("length")
              n108 = call-poly <vilib>:"Read Register.vi"("session in"=w469, "register address"=u32 1281 ("y"), "error in (no error)"=w470) -> ("session out"=w467:refnum<k21>, "data out"=w440:u64, "error out"=w468:errorcluster)  [unwired: 8 in, 2 out]
              n109 = Number To Boolean Array(number=w440) -> (Boolean array=w453:bool[])
              n110 = Tick Count (ms)() -> (millisecond timer value=w434:u32)
              n111 = Subtract(x=w434, y=w429) -> (x-y=w437:u32)
              n112 = Array Subset(array=w453, index=52, length=w459) -> (w454:bool[])
              n113 = Array Subset(array=w453, index=40, length=w459) -> (w452:bool[])
              n114 = Array Subset(array=w453, index=28, length=w459) -> (w451:bool[])
              n115 = Array Subset(array=w453, index=16, length=w459) -> (w450:bool[])
              n116 = Array Subset(array=w453, index=8, length=w458) -> (w449:bool[])
              n117 = Array Subset(array=w453, index=0, length=w458) -> (w448:bool[])
              n118 = Boolean Array To Number(Boolean array=w454) -> (number=w442:u16)
              n119 = Boolean Array To Number(Boolean array=w452) -> (number=w457:u16)
              n120 = Boolean Array To Number(Boolean array=w451) -> (number=w456:u16)
              n121 = Boolean Array To Number(Boolean array=w450) -> (number=w455:u16)
              n122 = Boolean Array To Number(Boolean array=w449) -> (number=w439:u8)
              "Command Cunter Feedback 6" <- w439
              n123 = Boolean Array To Number(Boolean array=w448) -> (number=→"Program Running Cunter 6":u8)
              n124 = Greater?(x=w437, y=u32 1000) -> (0:w432:bool)
              n125 = Build Array(w442, w457, w456, w455) -> (w443:u16[])
              n126 = Equal?(x=w430, y=w439) -> (x = y?=w438:bool)
              n127 = Subtract(x=w443, y=2048.0) -> (x-y=w446:dbl[])
              n128 = Or(x=w433, y=w432) -> (x .or. y?=w431:bool)
              n129 = Or(x=w432, y=w438) -> (x .or. y?=w435:bool)
              n130 = Divide(x=w446, y=204.8) -> (x/y=→"IP Feedback 6":dbl[])
            }
          }
          n131 = Wait Until Next ms Multiple(millisecond multiple=u32 100) -> ()  [unwired: 1 out]
        }
        n132 = Increment(x=w376) -> (x+1=w369:u8)
      }
    }
    frame 4 {
      n133 = for {
        tunnel: w478 -> [w492]
        tunnel: w476 -> [w491] mode=indexing
        shift-right: [w482] -> w473
        shift-left: w477 -> [w490]
        shift-right: [w488] -> w471
        shift-left: w480 -> [w487]
        tunnel: [w486] -> w474
        shift-right: [w483] -> w475
        shift-left: w479 -> [w485]
        tunnel: u8[] [204, 208, 212, 216] -> [w481] mode=indexing
        # "Change PID"
        n134 = Tick Count (ms)() -> (millisecond timer value=w484:u32)
        n135 = while {
          tunnel: w491 -> [w507]
          tunnel: w490 -> [w506]
          tunnel: [w505] -> w489
          tunnel: [w504] -> w488
          tunnel: w487 -> [w503]
          shift-right: [w497] -> _
          shift-left: w484 -> [w500]
          shift-right: [w495] -> w483
          shift-left: w485 -> [w501]
          tunnel: w481 -> [w494]
          tunnel: w492 -> [w508]
          tunnel: [w502] -> w486
          stop <- w498 stop-if-true
          n136 = flat-sequence {
            tunnel: w503 -> [w540]
            tunnel: w508 -> [w539]
            tunnel: [w519] -> w511
            tunnel: [w518] -> w510
            tunnel: [w516] -> w509
            tunnel: w507 -> [w517]
            tunnel: w506 -> [w516]
            tunnel: w501 -> [w514]
            tunnel: w500 -> [w515]
            tunnel: [w515] -> w499
            tunnel: [w514] -> w496
            tunnel: w494 -> [w513]
            tunnel: w511 -> [w583]
            tunnel: w510 -> [w582]
            tunnel: w509 -> [w543]
            tunnel: [w543] -> w505
            tunnel: [w581] -> w504
            tunnel: [w580] -> w502
            tunnel: w499 -> [w542]
            tunnel: [w548] -> w498
            tunnel: [w542] -> w497
            tunnel: w496 -> [w546]
            tunnel: [w544] -> w495
            frame #0 {
              w522 = u8 0  # 8 Bit Data 2
              w523 = u8 0  # 8 Bit Data 1
              n137 = To Single Precision Float(number=w517) -> (single precision float=w531:sgl)
              n138 = To Unsigned Byte Integer(number=w513) -> (unsigned 8bit integer=w512:u8)
              n139 = Type Cast(type=u32 0 ("index"), x=w531) -> (*(type *) &x=w524:u32)
              n140 = Number To Boolean Array(number=w522) -> (Boolean array=w520:bool[])
              n141 = Number To Boolean Array(number=w523) -> (Boolean array=w521:bool[])
              n142 = Number To Boolean Array(number=w516) -> (Boolean array=w526:bool[])
              n143 = Number To Boolean Array(number=w524) -> (Boolean array=w525:bool[])
              n144 = Number To Boolean Array(number=w512) -> (Boolean array=w535:bool[])
              n145 = Number To Boolean Array(number="CommandData 7") -> (Boolean array=w537:bool[])
              n146 = Replace Array Subset(array=w537, new element #1=w525, index #1=0 ("index"), new element #2=w520, index #2=32 ("index"), new element #3=w521, index #3=40 ("index"), new element #4=w526, index #4=48 ("index"), new element #5=w535, index #5=56 ("index")) -> (w536:bool[])
              n147 = Boolean Array To Number(Boolean array=w536) -> (number=w532:u64)
              n148 = call-poly <vilib>:"Write Register.vi"("session in"=w539, "register address"=u32 1538, "data"=w532, "error in (no error)"=w540) -> ("session out"=w518:refnum<k21>, "error out"=w519:errorcluster)  [unwired: 8 in, 2 out]
            }
            frame #1 {
              w571 = 8 ("length")
              w572 = 12 ("length")
              n149 = call-poly <vilib>:"Read Register.vi"("session in"=w582, "register address"=u32 1281 ("y"), "error in (no error)"=w583) -> ("session out"=w580:refnum<k21>, "data out"=w553:u64, "error out"=w581:errorcluster)  [unwired: 8 in, 2 out]
              n150 = Number To Boolean Array(number=w553) -> (Boolean array=w566:bool[])
              n151 = Tick Count (ms)() -> (millisecond timer value=w547:u32)
              n152 = Subtract(x=w547, y=w542) -> (x-y=w550:u32)
              n153 = Array Subset(array=w566, index=52, length=w572) -> (w567:bool[])
              n154 = Array Subset(array=w566, index=40, length=w572) -> (w565:bool[])
              n155 = Array Subset(array=w566, index=28, length=w572) -> (w564:bool[])
              n156 = Array Subset(array=w566, index=16, length=w572) -> (w563:bool[])
              n157 = Array Subset(array=w566, index=8, length=w571) -> (w562:bool[])
              n158 = Array Subset(array=w566, index=0, length=w571) -> (w561:bool[])
              n159 = Boolean Array To Number(Boolean array=w567) -> (number=w555:u16)
              n160 = Boolean Array To Number(Boolean array=w565) -> (number=w570:u16)
              n161 = Boolean Array To Number(Boolean array=w564) -> (number=w569:u16)
              n162 = Boolean Array To Number(Boolean array=w563) -> (number=w568:u16)
              n163 = Boolean Array To Number(Boolean array=w562) -> (number=w552:u8)
              "Command Cunter Feedback 7" <- w552
              n164 = Boolean Array To Number(Boolean array=w561) -> (number=→"Program Running Cunter 7":u8)
              n165 = Greater?(x=w550, y=u32 1000) -> (0:w545:bool)
              n166 = Build Array(w555, w570, w569, w568) -> (w556:u16[])
              n167 = Equal?(x=w543, y=w552) -> (x = y?=w551:bool)
              n168 = Subtract(x=w556, y=2048.0) -> (x-y=w559:dbl[])
              n169 = Or(x=w546, y=w545) -> (x .or. y?=w544:bool)
              n170 = Or(x=w545, y=w551) -> (x .or. y?=w548:bool)
              n171 = Divide(x=w559, y=204.8) -> (x/y=→"IP Feedback 7":dbl[])
            }
          }
          n172 = Wait Until Next ms Multiple(millisecond multiple=u32 100) -> ()  [unwired: 1 out]
        }
        n173 = Increment(x=w489) -> (x+1=w482:u8)
      }
    }
  }
  "com error out" <- w51
  n174 = case shown="10201" w42 {
    tunnel: w56 -> [w597 w608]
    tunnel: [w594 w607] -> w55
    tunnel: [w596 w606] -> w15
    tunnel: [w595 w605] -> w52
    tunnel: [w587 w606] -> w14
    tunnel: [w584 w605] -> w13
    frame 10201 {
      w590 = sgl 0.0 ("element")
      w592 = sgl 0.0 ("element")
      w593 = sgl 0.0 ("element")
      n175 = Index Array(array=w597, index #1=2 ("index"), index #2=5 ("index")) -> (element #1=w586:sgl, element #2=w585:sgl)
      n176 = Index Array(array=w597, index #1=1 ("index"), index #2=4 ("index")) -> (element #1=w589:sgl, element #2=w588:sgl)
      n177 = Index Array(array=w597, index #1=0 ("index"), index #2=3 ("index")) -> (element #1=w604:sgl, element #2=w591:sgl)
      n178 = Build Array "Enable"(w604, w590, w591, w590) -> (w594:sgl[])
      n179 = Build Array "R"(w586, w585) -> (w584:sgl[])
      n180 = Build Array "R"(w586, w592, w585, w592) -> (w595:sgl[])
      n181 = Build Array "IP"(w589, w588) -> (w587:sgl[])
      n182 = Build Array "IP"(w589, w593, w588, w593) -> (w596:sgl[])
    }
    frame 10401, Default {
      n183 = Index Array(array=w608, index #1=1 ("index"), index #2=4 ("index"), index #3=7 ("index"), index #4=10 ("index")) -> (element #1=w632:sgl, element #2=w627:sgl, element #3=w626:sgl, element #4=w625:sgl)
      n184 = Index Array(array=w608, index #1=0 ("index"), index #2=3 ("index"), index #3=6 ("index"), index #4=9 ("index")) -> (element #1=w616:sgl, element #2=w611:sgl, element #3=w610:sgl, element #4=w609:sgl)
      n185 = Index Array(array=w608, index #1=2 ("index"), index #2=5 ("index"), index #3=8 ("index"), index #4=11 ("index")) -> (element #1=w617:sgl, element #2=w622:sgl, element #3=w623:sgl, element #4=w624:sgl)
      n186 = Build Array "IP"(w632, w627, w626, w625) -> (w606:sgl[])
      n187 = Build Array "Enable"(w616, w611, w610, w609) -> (w607:sgl[])
      n188 = Build Array "R"(w617, w622, w623, w624) -> (w605:sgl[])
    }
  }
  n189 = To Word Integer(number=w52) -> (16bit integer=w54:i16[])
  n190 = To Byte Integer(number=dbl[] [0.0, 0.0, 0.0, 0.0] ("initialized array")) -> (8bit integer=w53:i8[])
  n191 = Greater Than 0?(x=w55) -> (x > 0?=w35:bool[])
  n192 = for {
    tunnel: w15 -> [w633] mode=indexing
    tunnel: w35 -> [w644] mode=indexing
    tunnel: w54 -> [w651] mode=indexing
    tunnel: w53 -> [w650] mode=indexing
    tunnel: [w640] -> w99 mode=indexing
    n193 = Number To Boolean Array(number=w651) -> (Boolean array=w646:bool[])
    n194 = Number To Boolean Array(number=w650) -> (Boolean array=w649:bool[])
    n195 = Multiply(x=3276.8, y=w633) -> (x*y=w634:dbl)
    n196 = Array Subset(array=w649, index=0, length=5) -> (w645:bool[])
    n197 = Replace Array Subset(array=w646, new element #1=w645, index #1=10 ("index"), new element #2=w644, index #2=15 ("index")) -> (w641:bool[])
    n198 = Add(x=32768.0, y=w634) -> (x+y=w637:dbl)
    n199 = To Unsigned Word Integer(number=w637) -> (unsigned 16bit integer=w638:u16)
    n200 = Boolean Array To Number(Boolean array=w641) -> (number=w639:u16)
    n201 = Join Numbers(hi=w638, lo=w639) -> ((hi.lo)=w640:u32)
  }
  n202 = Index Array(array=w99) -> (element #1=w100:u32, element #2=w102:u32, element #3=w101:u32, element #4=w103:u32)  [unwired: 4 in]
  n203 = Join Numbers(hi=w100, lo=w101) -> ((hi.lo)=w107:u64)
  n204 = Join Numbers(hi=w102, lo=w103) -> ((hi.lo)=w106:u64)
  n205 = call-poly <vilib>:"Write Register.vi"("session in"=w58, "register address"=u32 1536 ("y"), "data"=w107, "error in (no error)"=w59) -> ("session out"=w105:refnum<k21>, "error out"=w104:errorcluster)  [unwired: 8 in, 2 out]
  n206 = call-poly <vilib>:"Write Register.vi"("session in"=w105, "register address"=u32 1537 ("y"), "data"=w106, "error in (no error)"=w104) -> ("session out"=w57:refnum<k21>, "error out"=w60:errorcluster)  [unwired: 8 in, 2 out]
  n207 = call-poly <vilib>:"Read Register.vi"("session in"=w57, "register address"=u32 1280 ("y"), "error in (no error)"=w60) -> ("session out"=w62:refnum<k21>, "data out"=w90:u64, "error out"=w61:errorcluster)  [unwired: 8 in, 2 out]
  n208 = Split Number(x=w90) -> (hi(x)=w63:u32, lo(x)=w64:u32)
  n209 = Split Number(x=w63) -> (hi(x)=w65:u16, lo(x)=w66:u16)
  n210 = Split Number(x=w64) -> (hi(x)=w67:u16, lo(x)=w68:u16)
  n211 = call-poly <vilib>:"Read Register.vi"("session in"=w62, "register address"=u32 1281 ("y"), "error in (no error)"=w61) -> ("session out"=w31:refnum<k21>, "data out"=w70:u64, "error out"=w29:errorcluster)  [unwired: 8 in, 2 out]
  n212 = Build Array(w65, w66, w67, w68) -> (w69:u16[])
  n213 = for {
    tunnel: w69 -> [w654] mode=indexing
    tunnel: [w657] -> w38 mode=indexing
    tunnel: [w656] -> w39 mode=indexing
    tunnel: [w653] -> w34 mode=indexing
    tunnel: [w652] -> w40 mode=indexing
    n214 = Number To Boolean Array(number=w654) -> (Boolean array=w660:bool[])
    n215 = Array Subset(array=w660, index=8, length=7) -> (w659:bool[])
    n216 = Array Subset(array=w660, index=0, length=8) -> (w658:bool[])
    n217 = Array Subset(array=w660, index=15, length=1) -> (w655:bool[])
    n218 = Boolean Array To Number(Boolean array=w659) -> (number=w656:u8)
    n219 = Boolean Array To Number(Boolean array=w658) -> (number=w657:u8)
    n220 = Index Array(array=w655) -> (element=w653:bool)  [unwired: 1 in]
    n221 = Boolean To (0,1)(Boolean=w653) -> (0, 1=w652:i16)
  }
  "Status" <- w34
  "Heater DC Indicator" <- w39
  "Heater Frequency Indicator2" <- w38
  n222 = Number To Boolean Array(number=w70) -> (Boolean array=w83:bool[])
  n223 = Array Subset(array=w83, index=52, length=w77) -> (w82:bool[])
  n224 = Array Subset(array=w83, index=40, length=w77) -> (w84:bool[])
  n225 = Array Subset(array=w83, index=28, length=w77) -> (w85:bool[])
  n226 = Array Subset(array=w83, index=16, length=w77) -> (w86:bool[])
  n227 = Array Subset(array=w83, index=8, length=w78) -> (w87:bool[])
  n228 = Array Subset(array=w83, index=0, length=w78) -> (w88:bool[])
  n229 = Boolean Array To Number(Boolean array=w82) -> (number=w95:u16)
  n230 = Boolean Array To Number(Boolean array=w84) -> (number=w79:u16)
  n231 = Boolean Array To Number(Boolean array=w85) -> (number=w80:u16)
  n232 = Boolean Array To Number(Boolean array=w86) -> (number=w81:u16)
  n233 = Boolean Array To Number(Boolean array=w87) -> (number=→"Command Cunter Feedback":u8)
  n234 = Boolean Array To Number(Boolean array=w88) -> (number=→"Program Running Cunter":u8)
  n235 = Build Array(w95, w79, w80, w81) -> (w94:u16[])
  n236 = Subtract(x=w94, y=2048.0) -> (x-y=w92:dbl[])
  n237 = Divide(x=w92, y=204.8) -> (x/y=w37:dbl[])
  "IP Feedback" <- w37
  n238 = Unbundle By Name("SensorUsed") -> ("Sensor1"=w50:T4, "Sensor2"=w49:T4, "Sensor3"=w48:T4, "Sensor4"=w47:T4)
  n239 = Index Array(array=w37) -> (element=→"element":dbl)  [unwired: 1 in]
  n240 = Not Equal?(x=w35, y=w34) -> (x != y?=w33:bool[])
  n241 = Or Array Elements(Boolean array=w33) -> (logical OR=w28:bool)
  n242 = Build Array(w50, w49, w48, w47) -> (w46:T5)
  n243 = for {
    tunnel: w46 -> [w672] mode=indexing
    tunnel: [w668] -> w41 mode=indexing
    tunnel: w37 -> [w667] mode=indexing
    n244 = Unbundle By Name(w672) -> ("Lambda"=w670:dbl[], "Ip"=w669:dbl[], "Enable mA"=w671:bool)
    n245 = case shown="False" w671 {
      tunnel: w667 -> [w676 w678]
      tunnel: [w675 w678] -> w668
      tunnel: w670 -> [w674 _]
      tunnel: w669 -> [w673 _]
      frame False {
        n246 = Threshold 1D Array(2:w676, 3:w673) -> (0:w677:dbl)  [unwired: 1 in]
        n247 = Interpolate 1D Array(1:w677, 2:w674) -> (0:w675:dbl)
      }
      frame True {
      }
    }
  }
  n248 = case shown="False" w28 {
    tunnel: [w679 w680] -> w32
    frame False {
      w679 = 2  # verde
    }
    frame True {
      w680 = 1  # rosso
    }
  }
  n249 = call-poly <vilib>:"Set Device Property.vi"("session in"=w31, "property"=refnum<k21> "AA.ReadyLedColor", "property value"=w32, "error in (no error)"=w29) -> ("session out"=w21:refnum<k21>, "error out"=w22:errorcluster)  [unwired: 10 in]
  n250 = Concatenate Strings("devices 2") -> (w20:string)
  n251 = call <vilib>:"Commit Properties (Generic).vi"("session in"=w21, "resources"=w20, "error in (no error)"=w22) -> ("session out"=→"session out":refnum<k21>, "error out"=w3:errorcluster)  [unwired: 11 in]
  "error out" <- w3
  n252 = Multiply(x=1.0, y=w14) -> (x*y=w24:dbl[])
  n253 = Divide(x=470.0, y=w13) -> (x/y=w16:dbl[])
  n254 = Add(x=5.0, y=w24) -> (x+y=w17:dbl[])
  n255 = To Single Precision Float(number=w16) -> (single precision float=w11:sgl[])
  n256 = To Single Precision Float(number=w17) -> (single precision float=w12:sgl[])
  n257 = To Single Precision Float(number=w14) -> (single precision float=w10:sgl[])
  n258 = To Single Precision Float(number=w13) -> (single precision float=w9:sgl[])
  n259 = case shown="10201" w42 {
    tunnel: [w681 w702] -> w6
    tunnel: w41 -> [w701 w710]
    tunnel: w40 -> [w692 w709]
    tunnel: w39 -> [w691 w708]
    tunnel: w38 -> [w690 w707]
    tunnel: w10 -> [w685 w706]
    tunnel: w9 -> [w684 w705]
    tunnel: w12 -> [w683 w704]
    tunnel: w11 -> [w682 w703]
    frame 10201 {
      n260 = Index Array(array=w701) -> (element #1=w700:dbl, element #3=w699:dbl)  [unwired: 3 in, 1 out]
      n261 = Index Array(array=w692) -> (element #1=w697:i16, element #3=w698:i16)  [unwired: 3 in, 1 out]
      n262 = Index Array(array=w691) -> (element #1=w696:u8, element #3=w695:u8)  [unwired: 3 in, 1 out]
      n263 = Index Array(array=w690) -> (element #1=w693:u8, element #3=w694:u8)  [unwired: 3 in, 1 out]
      n264 = Build Array(w700, w699) -> (w689:dbl[])
      n265 = Build Array(w697, w698) -> (w688:i16[])
      n266 = Build Array(w696, w695) -> (w687:u8[])
      n267 = Build Array(w693, w694) -> (w686:u8[])
      n268 = Interleave 1D Arrays(w689, w688, w687, w686, w685, w684, w683, w682) -> (w681:dbl[])
    }
    frame 10401, Default {
      n269 = Interleave 1D Arrays(w710, w709, w708, w707, w706, w705, w704, w703) -> (w702:dbl[])
    }
  }
  n270 = Unbundle By Name(w3) -> ("code"=w1:i32)
  n271 = Build Array (concatenate)(w6, "period", w1) -> (w4:dbl[])
  n272 = Replace Array Subset(array="VS feedback", new element=w4, index=0) -> (→"VS feedback":dbl[])
